vi "calculateRangeModePositions.vi"(6 "Delay between send and receive [ms]":i32=100, 8 "error in (no error)":errorcluster, 10 "calculateRangeModePositions":T1, 11 "CCD in":refnum<class "CCD.lvclass">) -> (0 "error out":errorcluster, 1 "ID":i32, 2 "results-JSON string":string, 3 "CCD out":refnum<class "CCD.lvclass">)   [LabVIEW 2023, in "CCD.lvclass"]
doc: "tarts an acquisition that has been set up according to the previously defined acquisition parameters.\n\nNote: To specify the acquisition parameters please see ccd_setROI and ccd_setXAxisConversionType. If there are no acquisition parameters specified at the time of acquisition it may result in no data being generated."
uses:
  CCD.lvclass
  CCD.lvclass/CCD.ctl
  20f7d3bd-08ac-4524-9bed-df36c1da25a0.vi
  GenericDevice/GenericDevice.lvclass
  cab240a6-cbf4-4e2c-ab79-96d9c1b88265.vi
  6968c003-a3a8-4fe6-bd53-13ad12dc6eda.vi
  d8999305-94e7-4d24-b768-1afaedf83813.vi
  4fd64012-a7af-4048-b972-7cd663129ff9.vi
  <vilib>/JDP Science/JSONtext/JSONtext.lvlib
panel:
  # "Connector Pane"
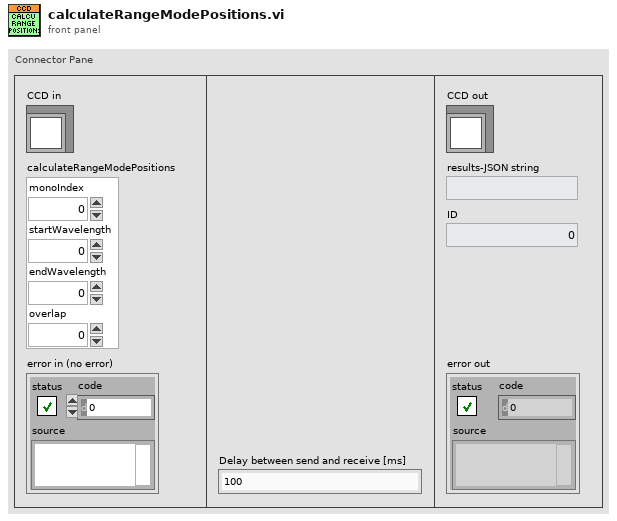
[diagram p1: front panel]
types:
  T1 = cluster{"monoIndex":i32, "startWavelength":dbl, "endWavelength":dbl, "overlap":dbl}
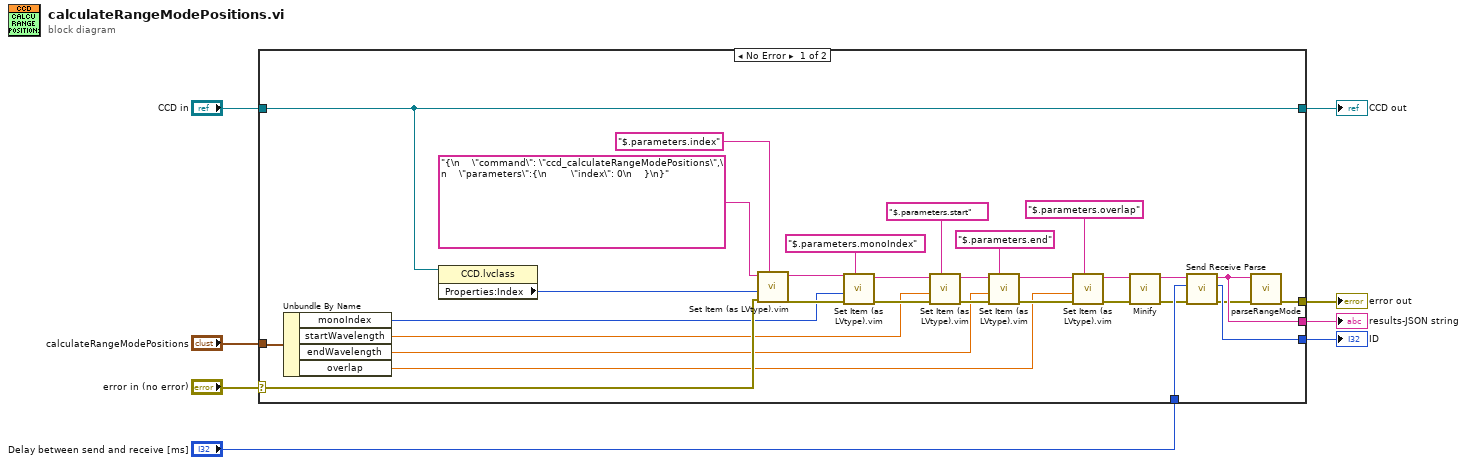
[diagram p0: block diagram]
diagram:
  n1 = case shown="No Error" "error in (no error)" {
    selector: "error in (no error)" -> [w35 w41]
    tunnel: [w12 w41] -> w7
    tunnel: [w37 w40] -> w5
    tunnel: "CCD in" -> [w37 w40]
    tunnel: [w14 _] -> w4
    tunnel: [w30 _] -> w3
    tunnel: "Delay between send and receive [ms]" -> [w29 _]
    tunnel: "calculateRangeModePositions" -> [w28 _]
    frame No Error {
      n2 = Unbundle By Name(w28) -> ("monoIndex"=w18:i32, "startWavelength"=w17:dbl, "endWavelength"=w16:dbl, "overlap"=w15:dbl)
      n3 = property class="CCD.lvclass"(reference=w37) -> ("Properties:Index"=w36:i32)  [unwired: 1 in, 2 out]
      n4 = call "Set Item (as LVtype).vim"("$Path or Item Name"="$.parameters.index", "error in (no error)"=w35, "Anything"=w36, "JSON"="{\n    \"command\": \"ccd_calculateRangeModePositions\",\n    \"parameters\":{\n        \"index\": 0\n    }\n}") -> ("error out"=w33:errorcluster, "<JSON>"=w31:string)  [unwired: 4 in, 1 out]
      n5 = call "Set Item (as LVtype).vim"("$Path or Item Name"="$.parameters.monoIndex", "error in (no error)"=w33, "Anything"=w18, "JSON"=w31) -> ("error out"=w32:errorcluster, "<JSON>"=w26:string)  [unwired: 4 in, 1 out]
      n6 = call "Set Item (as LVtype).vim"("$Path or Item Name"="$.parameters.start", "error in (no error)"=w32, "Anything"=w17, "JSON"=w26) -> ("error out"=w27:errorcluster, "<JSON>"=w23:string)  [unwired: 4 in, 1 out]
      n7 = call "Set Item (as LVtype).vim"("$Path or Item Name"="$.parameters.end", "error in (no error)"=w27, "Anything"=w16, "JSON"=w23) -> ("error out"=w24:errorcluster, "<JSON>"=w20:string)  [unwired: 4 in, 1 out]
      n8 = call "Set Item (as LVtype).vim"("$Path or Item Name"="$.parameters.overlap", "error in (no error)"=w24, "Anything"=w15, "JSON"=w20) -> ("error out"=w21:errorcluster, "<JSON>"=w10:string)  [unwired: 4 in, 1 out]
      n9 = call <vilib>:"Minify.vi"("error in (no error)"=w21, "JSON"=w10) -> ("error out"=w11:errorcluster, "<JSON>"=w9:string)  [unwired: 7 in, 1 out]
      n10 = call "Send Receive Parse.vi"("error in"=w11, "Delay between send and receive [ms]"=w29, "<JSON>"=w9) -> ("error out"=w13:errorcluster, "ID"=w30:i32, "results-JSON string"=w14:string)  [unwired: 6 in]
      n11 = call "parseRangeMode.vi"("error in (no error)"=w13, "String"=w14) -> ("error out"=w12:errorcluster)  [unwired: 8 in, 1 out]
    }
    frame Error {
    }
  }
  "error out" <- w7
  "CCD out" <- w5
  "results-JSON string" <- w4
  "ID" <- w3
